vi "Y_profile_adjustable.vi"(1 "Vy min(bits)":i16, 2 "no. of lines until end of fly-back":u16, 3 "line counter":u16, 4 "no. of lines until start of fly-back":u16, 5 "y amplitude":u16, 6 "y step size":u16, 7 "y acquire? (line counter<number of lines)":bool) -> (0 "y signal":i16)   [LabVIEW 2010]
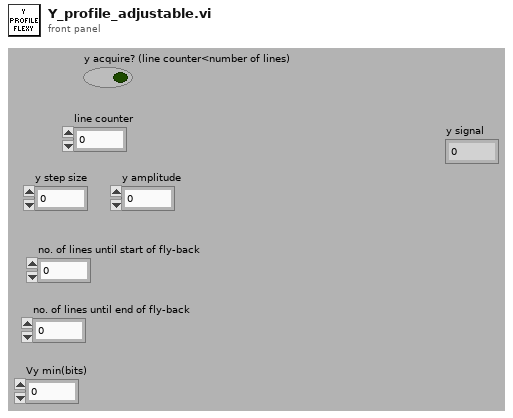
[diagram p1: front panel]
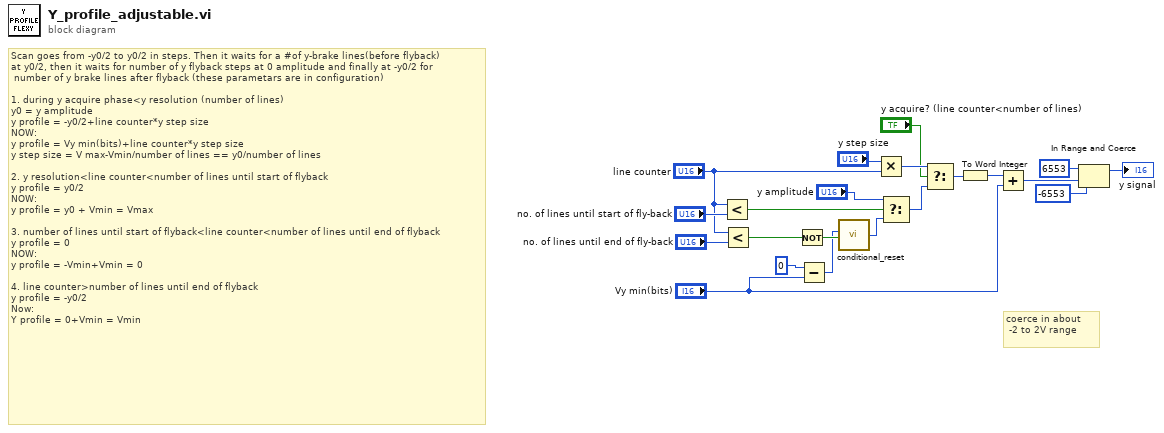
[diagram p0: block diagram]
diagram:
  # "coerce in about\n -2 to 2V range"
  # "Scan goes from -y0/2 to y0/2 in steps. Then it waits for a #of y-brake lines(before flyback) \nat y0/2, then it waits for number of y flyback steps at 0 amplitude and finally at -y0/2 for\n number of y brake lines after flyback (these parametars are in configuration)\n\n1. during y acquire phase<y resolution (number of lines)\ny0 = y amplitude\ny profile = -y0/2+line counter*y step size\nNOW:\ny profile = Vy min(bits)+line counter*y step size\ny step size = V max-Vmin/number of lines == y0/number of lines\n\n2. y resolution<line counter<number of lines until start of flyback\ny profile = y0/2\nNOW:\ny profile = y0 + Vmin = Vmax\n\n3. number of lines until start of flyback<line counter<number of lines until end of flyback\ny profile = 0\nNOW:\ny profile = -Vmin+Vmin = 0\n\n4. line counter>number of lines until end of flyback\ny profile = -y0/2\nNow:\nY profile = 0+Vmin = Vmin"
  n1 = Less?(x="line counter", y="no. of lines until start of fly-back") -> (x < y?=w15:bool)
  n2 = Less?(x="line counter", y="no. of lines until end of fly-back") -> (x < y?=w17:bool)
  n3 = Not(x=w17) -> (.not. x?=w20:bool)
  n4 = Subtract(x=i16 0, y="Vy min(bits)") -> (x-y=w4:i16)
  n5 = call "conditional_reset.vi"("reset?"=w20, "number in"=w4) -> ("number out"=w12:u16)  [unwired: 4 in]
  n6 = Multiply(x="y step size", y="line counter") -> (x*y=w16:u16)
  n7 = Select(t="y amplitude", s=w15, f=w12) -> (s? t:f=w13:u16)
  n8 = Select(t=w16, s="y acquire? (line counter<number of lines)", f=w13) -> (s? t:f=w19:u16)
  n9 = To Word Integer(number=w19) -> (16bit integer=w10:i16)
  n10 = Add(x=w10, y="Vy min(bits)") -> (x+y=w8:i16)
  n11 = In Range and Coerce(upper limit=i16 6553, x=w8, lower limit=i16 -6553) -> (coerced(x)=→"y signal":i16)  [unwired: 1 out]
